vi "IPC-Modbus-Transfer-DecodeRequest-WriteMulCoils.vi"(4 "无符号字节数组":u8[](array[numeric])) -> (1 "Write Multiple Coils request":T1)   [LabVIEW 2014]
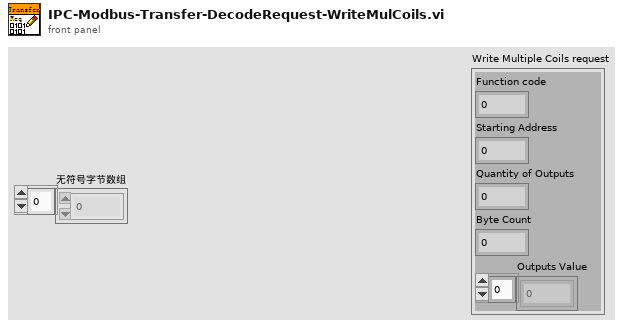
[diagram p1: front panel]
types:
  T1 = cluster{"Function code":u8, "Starting Address":u16, "Quantity of Outputs":u16, "Byte Count":u8, "Outputs Value":u8[]}
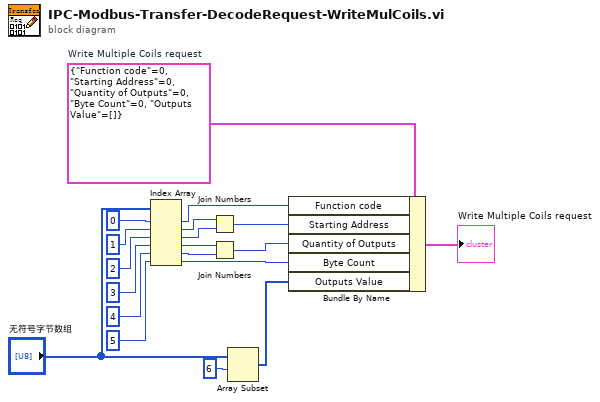
[diagram p0: block diagram]
diagram:
  w19 = T1 {"Function code"=0, "Starting Address"=0, "Quantity of Outputs"=0, "Byte Count"=0, "Outputs Value"=[]}  # Write Multiple Coils request
  n1 = Index Array(array="无符号字节数组", index #1=0 ("索引"), index #2=1 ("索引"), index #3=2 ("索引"), index #4=3 ("索引"), index #5=4 ("索引"), index #6=5 ("索引")) -> (element #1=w13:u8, element #2=w12:u8, element #3=w11:u8, element #4=w9:u8, element #5=w8:u8, element #6=w6:u8)
  n2 = Join Numbers(hi=w12, lo=w11) -> ((hi.lo)=w10:u16)
  n3 = Join Numbers(hi=w9, lo=w8) -> ((hi.lo)=w7:u16)
  n4 = Array Subset(array="无符号字节数组", index=6 ("索引")) -> (w2:u8[])  [unwired: 1 in]
  n5 = Bundle By Name(cluster=w19, "Function code"=w13, "Starting Address"=w10, "Quantity of Outputs"=w7, "Byte Count"=w6, "Outputs Value"=w2) -> (→"Write Multiple Coils request":T1)
